vi "Panel_Control.vi"() -> ()   [LabVIEW 2024]
panel:
  in  "p":bool
  in  "Set_Velocidad 4":bool
  in  "Set_Velocidad 3":bool
  in  "Set_Velocidad 2":bool
  out "Izquierda":bool
  out "Derecha":bool
  in  "Cantidad Vueltas":dbl
  in  "Set_Home 2":bool
  in  "Velocidad_Definida":i16(slide) scale=0.0..3000.0
  out "Velocimetro":dbl(knob) scale=0.0..3000.0
  in  "Switch_Motor":bool
  out "Activación_Motor":bool
  in  "Set_Velocidad":bool
  out "Numeric":dbl
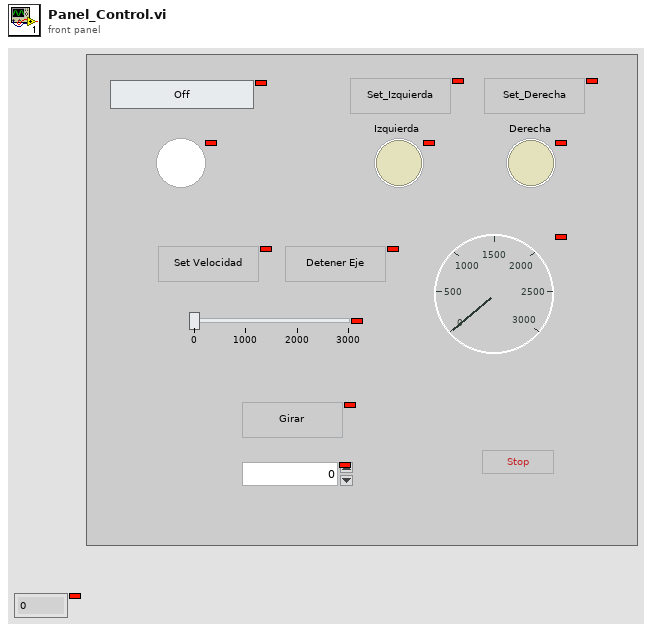
[diagram p1: front panel]
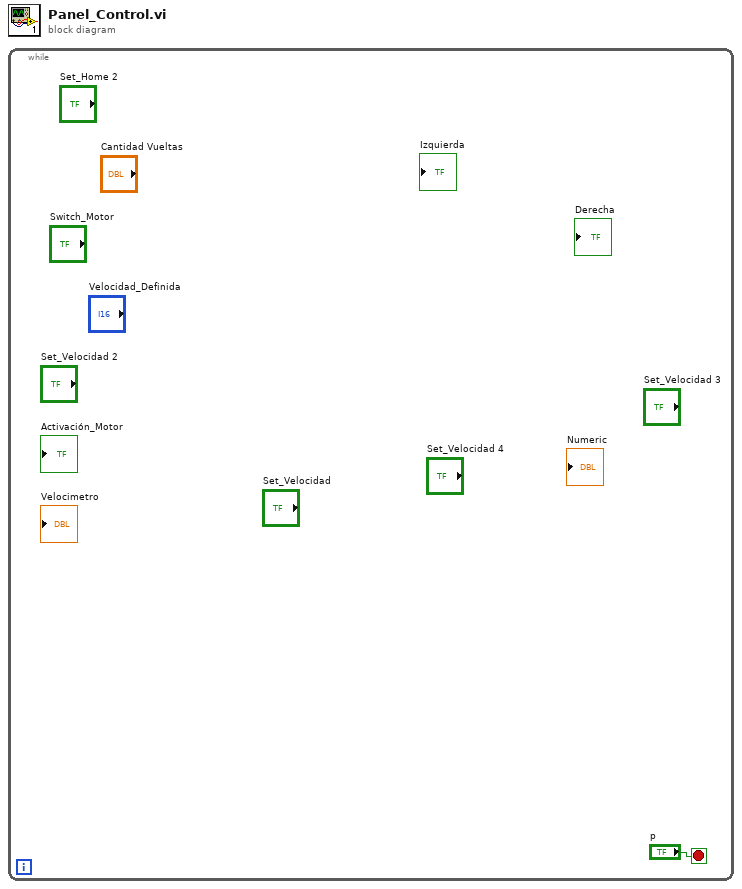
[diagram p0: block diagram]
diagram:
  n1 = while {
    stop <- "p" stop-if-true
  }
